vi "Controller Handlers.vi"(9 "Controller Handler Map":T1, 10 "Controller in":refnum<class "Controller.lvclass">, 11 "Processing In":refnum<class "Processing.lvclass">) -> (0 "error out":errorcluster, 2 "Controller":refnum<class "Controller.lvclass">, 3 "Processing":refnum<class "Processing.lvclass">)   [LabVIEW 2020, in "HTTP Server.lvlib" / "Server.lvclass"]
uses:
  Server.lvclass
  Server.lvclass/Server.ctl
  Processing Step.ctl
  HTTP Server.lvlib
  Processing/Processing.lvclass
  Controller Handler/Controller Handler.lvclass
  C:/dev/lv20CE/relink/lv-http-server/HTTP Server/Controller Handler/Controller Handler.lvclass
  C:/dev/lv20CE/relink/lv-http-server/HTTP Server/Handler/Handler.lvclass
  Priority.ctl
  Controller Handler Map.ctl
  Controller/Controller.lvclass
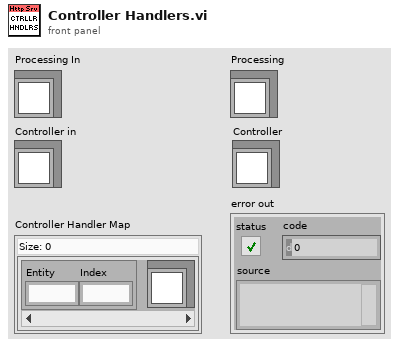
[diagram p1: front panel]
types:
  T1 = typedef "HTTP Server.lvlib/Controller Handler Map.ctl" = map{T2, refnum<class "Controller Handler.lvclass">}
  T2 = typedef "HTTP Server.lvlib/Priority.ctl" = cluster{"Entity":u16, "Index":u16}
  T3 = typedef "HTTP Server.lvlib/Processing Step.ctl" = enum16{"Connection", "Request", "Routing", "Controller Init", "Controller", "Response", "Complete", "Exception"}
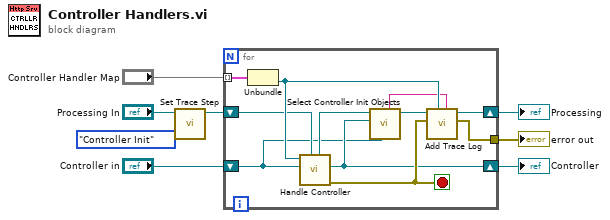
[diagram p0: block diagram]
diagram:
  n1 = call "Set Trace Step.vi"("Processing Step"=Processing_Step."Controller Init", "Processing in"="Processing In") -> ("Processing out"=w6:refnum<class "Processing.lvclass">)  [unwired: 9 in]
  n2 = for {
    tunnel: "Controller Handler Map" -> [w19] mode=indexing
    shift-right: [w18] -> w5
    shift-left: w6 -> [w11]
    tunnel: [w13] -> w4
    shift-right: [w12] -> w1
    shift-left: "Controller in" -> [w9]
    stop <- w16 stop-if-true
    n3 = Unbundle(w19) -> ("Handler"=w17:refnum<class "Controller Handler.lvclass">)  [unwired: 1 out]
    n4 = call-dynamic "Handle Controller.vi"("Processing In"=w11, "Controller in"=w9, "Arguments Handler in"=w17) -> ("error out"=w16:errorcluster, "Controller"=w12:refnum<class "Controller.lvclass">, "Processing"=w15:refnum<class "Processing.lvclass">)  [unwired: 6 in]
    n5 = call "Select Controller Init Objects.vi"("Initial Controller"=w9, "Controller"=w12, "Inputs"=w15) -> ("Updated Inputs"=w14:refnum<class "Processing.lvclass">, "Trace Message"=w10:string)  [unwired: 7 in]
    n6 = call "Add Trace Log.vi"("Info"=w10, "LabVIEW Object"=w17, "error in (no error)"=w16, "Processing in"=w14) -> ("error out"=w13:errorcluster, "Processing out"=w18:refnum<class "Processing.lvclass">)  [unwired: 6 in]
  }
  "Processing" <- w5
  "error out" <- w4
  "Controller" <- w1
